vi "AgPSA _Init and Setup Single Sweep SpecAn.vi"(10 "Ref Level":i32, 11 "VISA resource name":refnum<visa-resource-name>="SpecAn_1") -> (0 "error out":errorcluster, 3 "VISA resource name out":refnum<visa-resource-name>)   [LabVIEW 2015]
uses:
  <instrlib>/Agilent MXA Series/Public/Configure/Marker/Configure Marker Type (Swept SA).vi
  <instrlib>/Agilent MXA Series/Agilent MXA Series.lvlib
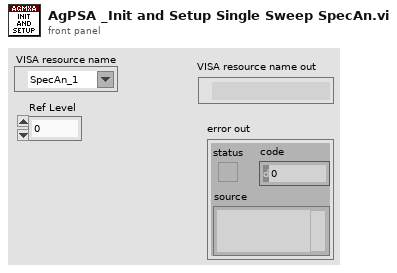
[diagram p1: front panel]
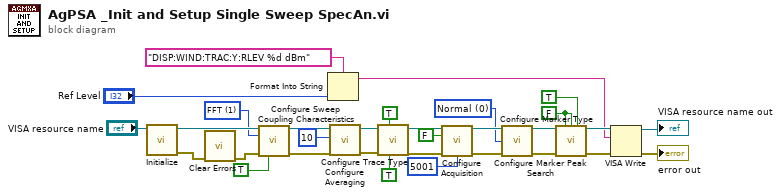
[diagram p0: block diagram]
diagram:
  w12 = 1 items=["Auto", "FFT", "Sweep"] ("Sweep Type (0: Auto)")
  w16 = FALSE ("Enable Peak Excursion (T: Enable)")
  w20 = 0 items=["Normal", "Delta", "Fixed", "Off"] ("Marker Type (0: Normal)")
  n1 = call <instrlib>:"Initialize.vi"("VISA resource name"="VISA resource name") -> ("error out"=w15:errorcluster, "VISA resource name out"=w14:refnum<visa-resource-name>)  [unwired: 9 in]
  n2 = call <vilib>:"Clear Errors.vi"("error in (no error)"=w15) -> ("error out"=w13:errorcluster)  [unwired: 5 in, 1 out]
  n3 = call <instrlib>:"Configure Sweep Coupling Characteristics.vi"("VISA resource name"=w14, "Sweep Type (0: Auto)"=w12, "error in (no error)"=w13, "Auto SPAN/RBW Ratio (T: Enable)"=TRUE) -> ("VISA resource name out"=w11:refnum<visa-resource-name>, "error out"=w10:errorcluster)  [unwired: 10 in]
  n4 = Format Into String(format string="DISP:WIND:TRAC:Y:RLEV %d dBm", "Ref Level") -> (resulting string=w1:string)  [unwired: 2 in, 1 out]
  n5 = call <instrlib>:"Configure Averaging.vi"("error in (no error)"=w10, "Average Count (100)"=10, "VISA resource name"=w11) -> ("error out"=w26:errorcluster, "VISA resource name out"=w28:refnum<visa-resource-name>)  [unwired: 7 in]
  n6 = call <instrlib>:"Configure Trace Type.vi"("Enable Trace Display (F: Disable)"=TRUE, "Enable Trace Update (F: Disable)"=TRUE, "error in (no error)"=w26, "VISA resource name"=w28) -> ("error out"=w25:errorcluster, "VISA resource name out"=w27:refnum<visa-resource-name>)  [unwired: 6 in]
  n7 = call <instrlib>:"Configure Acquisition.vi"("VISA resource name"=w27, "Enable Continuous Sweep (T: Enable)"=FALSE, "error in (no error)"=w25, "Sweep Points (1001)"=5001) -> ("VISA resource name out"=w22:refnum<visa-resource-name>, "error out"=w21:errorcluster)  [unwired: 10 in]
  n8 = call-poly <instrlib>:"Configure Marker Type.vi"("VISA resource name"=w22, "Marker Type (0: Normal)"=w20, "error in (no error)"=w21) -> ("VISA resource name out"=w19:refnum<visa-resource-name>, "error out"=w18:errorcluster)  [unwired: 11 in]
  n9 = call <instrlib>:"Configure Marker Peak Search.vi"("VISA resource name"=w19, "Enable Peak Excursion (T: Enable)"=w16, "Enable Peak Threshold (T: Enable)"=w16, "Enable Continuous Peak Search (F: Disable)"=TRUE, "error in (no error)"=w18) -> ("VISA resource name out"=w5:refnum<visa-resource-name>, "error out"=w7:errorcluster)  [unwired: 9 in]
  n10 = VISA Write(VISA resource name=w5, write buffer=w1, error in (no error)=w7) -> (VISA resource name out=→"VISA resource name out":refnum<visa-resource-name>, error out=→"error out":errorcluster)  [unwired: 1 out]
